vi "Create Opaque Structs.vi"(4 "Manifestation Ancestor":refnum<vi>, 9 "Opaque Structs":T1[](array[typedef]), 10 "Existing Class Ref Map":variant, 11 "Owning LVLib":refnum<vi>) -> (2 "Augmented Class Ref Map":variant, 3 "Owning LVLib Dup":refnum<vi>)   [LabVIEW 2013]
uses:
  Data Structures/JSON/Class.ctl
  Data Structures/JSON/Enum.ctl
  Data Structures/JSON/Enum Value.ctl
  Data Structures/JSON/Method.ctl
  Data Structures/JSON/Param.ctl
  Data Structures/JSON/Connector Pane.ctl
  Data Structures/JSON/Connector Pane Terminal.ctl
  Data Structures/JSON/Property.ctl
  Param Writers/TypeConv/Action.ctl
  Param Writers/TypeConv/Category.ctl
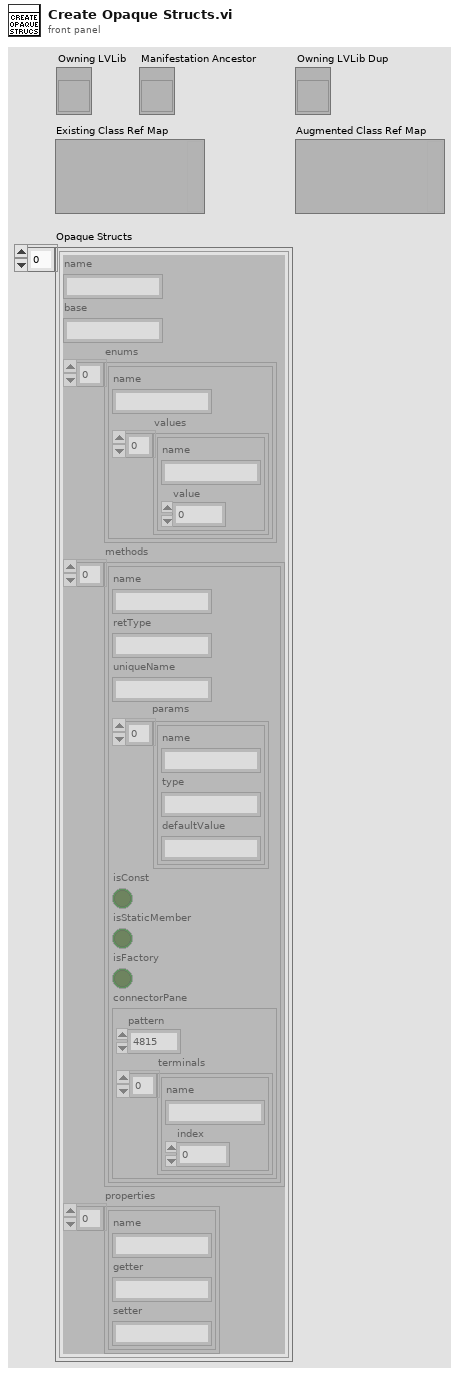
[diagram p1: front panel]
types:
  T1 = typedef "Class.ctl" = cluster{"name":string, "base":string, "enums":T2[], "methods":T4[], "properties":T8[]}
  T2 = typedef "Enum.ctl" = cluster{"name":string, "values":T3[]}
  T3 = typedef "Enum Value.ctl" = cluster{"name":string, "value":i32}
  T4 = typedef "Method.ctl" = cluster{"name":string, "retType":string, "uniqueName":string, "params":T5[], "isConst":bool, "isStaticMember":bool, "isFactory":bool, "connectorPane":T6}
  T5 = typedef "Param.ctl" = cluster{"name":string, "type":string, "defaultValue":string}
  T6 = typedef "Connector Pane.ctl" = cluster{"pattern":u32, "terminals":T7[]}
  T7 = typedef "Connector Pane Terminal.ctl" = cluster{"name":string, "index":u32}
  T8 = typedef "Property.ctl" = cluster{"name":string, "getter":string, "setter":string}
  T9 = typedef "Category.ctl" = enum16{"Invalid", "Void", "Boolean", "Numeric", "Enum", "SimpleStruct", "OpaqueStruct", "SimpleIdentity", "QObject", "SimpleContainer", "FullArray"}
  T10 = typedef "Action.ctl" = enum16{"Register Type", "Register Projection", "Obtain Writer", "Get Projection", "Get Type Path", "Get Type Category"}
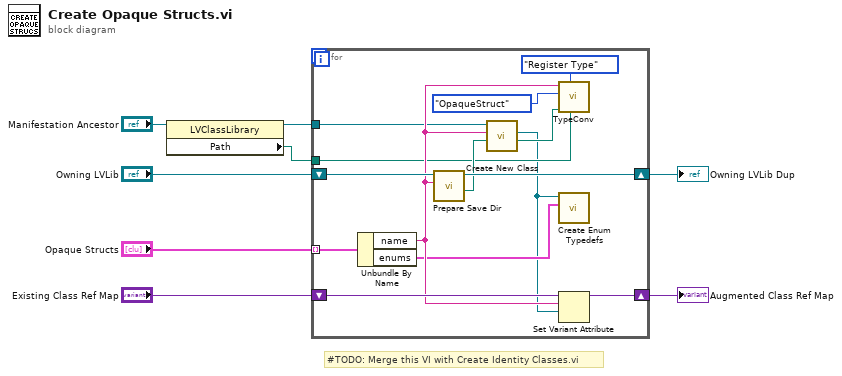
[diagram p0: block diagram]
diagram:
  # "#TODO: Merge this VI with Create Identity Classes.vi"
  n1 = property class="LVClassLibrary"(reference="Manifestation Ancestor") -> (reference out=w2:refnum<vi>, "Path"=w1:path)  [unwired: 1 in, 1 out]
  n2 = for {
    tunnel: "Opaque Structs" -> [w15] mode=indexing
    shift-right: [w20] -> w7
    shift-left: "Owning LVLib" -> [w19]
    shift-right: [w16] -> w6
    shift-left: "Existing Class Ref Map" -> [w17]
    tunnel: w2 -> [w12]
    tunnel: w1 -> [w10]
    n3 = Unbundle By Name(w15) -> ("name"=w14:string, "enums"=w13:T2[])
    n4 = call "Prepare Save Dir.vi"("Entity Name"=w14, "Owning LVLib"=w19) -> ("Entity Path"=w18:path, "Owning LVLib Dup"=w20:refnum<vi>)  [unwired: 8 in]
    n5 = call "Create New Class.vi"("Class Path"=w18, "Class Name"=w14, "Base Class"=w12) -> ("Class Path Dup"=w11:path, "New Class"=w9:refnum<vi>)  [unwired: 7 in]
    n6 = call "TypeConv.vi"("Manifestation Ancestor Path"=w10, "Action"=Action."Register Type", "Type Path"=w11, "Category"=Category."OpaqueStruct", "Type Name"=w14) -> ()  [unwired: 2 in, 5 out]
    n7 = call "Create Enum Typedefs.vi"("Enums"=w13, "Owning Lib"=w9) -> ()  [unwired: 9 in, 1 out]
    n8 = Set Variant Attribute(Variant=w17, name=w14, value=w9) -> (Variant out=w16:variant)  [unwired: 1 in, 2 out]
  }
  "Owning LVLib Dup" <- w7
  "Augmented Class Ref Map" <- w6
